vi "Get_PSU_Limits.vi"(8 "error in (no error)":errorcluster) -> (0 "error out":errorcluster, 3 "Limits":T1 {"High Voltage" format="%#_4g"})   [LabVIEW 2015]
uses:
  Limits_In.ctl
  <vilib>/addons/database/_DB Variant To Data/Database Variant To Data.xnode
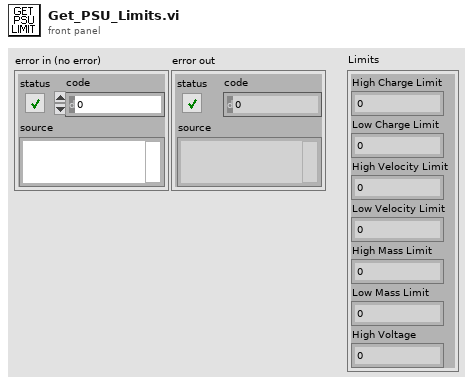
[diagram p1: front panel]
types:
  T1 = typedef "Limits_In.ctl" = cluster{"High Charge Limit":fxp<+,22,-41>, "Low Charge Limit":fxp<+,22,-41>, "High Velocity Limit":fxp<+,18,18>, "Low Velocity Limit":fxp<+,18,18>, "High Mass Limit":fxp<+,32,-37>, "Low Mass Limit":fxp<+,32,-37>, "High Voltage":fxp<+,15,22>}
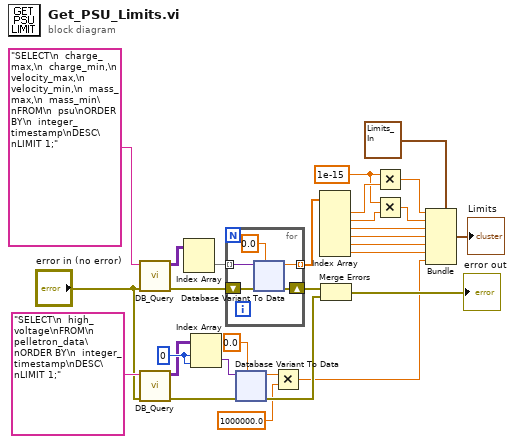
[diagram p0: block diagram]
diagram:
  w1 = 1e-15 ("x")
  w22 = 0 ("index (row)")
  n1 = call "DB_Query.vi"("error in (no error)"="error in (no error)", "Parameterized Query"="SELECT\n  charge_max,\n  charge_min,\n  velocity_max,\n  velocity_min,\n  mass_max,\n  mass_min\nFROM\n  psu\nORDER BY\n  integer_timestamp\nDESC\nLIMIT 1;") -> ("error out"=w27:errorcluster, "Results"=w28:variant[][])  [unwired: 7 in, 1 out]
  n2 = call "DB_Query.vi"("error in (no error)"="error in (no error)", "Parameterized Query"="SELECT\n  high_voltage\nFROM\n  pelletron_data\nORDER BY\n  integer_timestamp\nDESC\nLIMIT 1;") -> ("error out"=w19:errorcluster, "Results"=w21:variant[][])  [unwired: 7 in, 1 out]
  n3 = Index Array(array=w28) -> (element=w12:variant[])  [unwired: 2 in]
  n4 = Index Array(array=w21, index (row)=w22, index (col)=w22) -> (element=w18:variant)
  n5 = for {
    tunnel: w12 -> [w33] mode=indexing
    shift-right: [w32] -> w25
    shift-left: w27 -> [w34]
    tunnel: [w30] -> w11 mode=indexing
    n6 = xnode "Database Variant To Data"("database variant"=w33, "error in (no error)"=w34, "type"=0.0 ("length")) -> ("data"=w30:dbl, "error out"=w32:errorcluster)
  }
  n7 = xnode "Database Variant To Data"("database variant"=w18, "error in (no error)"=w19, "type"=0.0 ("length")) -> ("data"=w16:dbl, "error out"=w17:errorcluster)
  n8 = Multiply(x=w16, y=1000000.0 ("x")) -> (x*y=w6:dbl)
  n9 = Index Array(array=w11) -> (element #1=w5:dbl, element #2=w4:dbl, element #3=w7:dbl, element #4=w8:dbl, element #5=w9:dbl, element #6=w10:dbl)  [unwired: 6 in]
  n10 = Merge Errors(w25, w17) -> (→"error out":errorcluster)
  n11 = Multiply(x=w1, y=w5) -> (x*y=w2:dbl)
  n12 = Multiply(x=w1, y=w4) -> (x*y=w3:dbl)
  n13 = Bundle(cluster=T1 {"High Charge Limit"=0.0, "Low Charge Limit"=0.0, "High Velocity Limit"=0.0, "Low Velocity Limit"=0.0, "High Mass Limit"=0.0, "Low Mass Limit"=0.0, "High Voltage"=0.0} ("Limits"), "High Charge Limit"=w2, "Low Charge Limit"=w3, "High Velocity Limit"=w7, "Low Velocity Limit"=w8, "High Mass Limit"=w9, "Low Mass Limit"=w10, "High Voltage"=w6) -> (→"Limits":T1)
